vi "Initialize.vi"(8 "error in (no error)":errorcluster, 10 "config path":path, 11 "ThAr in":refnum<class "ThAr.lvclass">) -> (0 "error out":errorcluster, 3 "ThAr out":refnum<class "ThAr.lvclass">)   [LabVIEW 2016, in "ThAr.lvclass"]
uses:
  ThAr.lvclass
  <vilib>/Utility/config.llb/Read Key (Double).vi
  <vilib>/Utility/config.llb/Read Key (U32).vi
  <vilib>/Utility/config.llb/Read Key (String).vi
  Lamp.lvclass
  <vilib>/Utility/config.llb/NI_LVConfig.lvlib
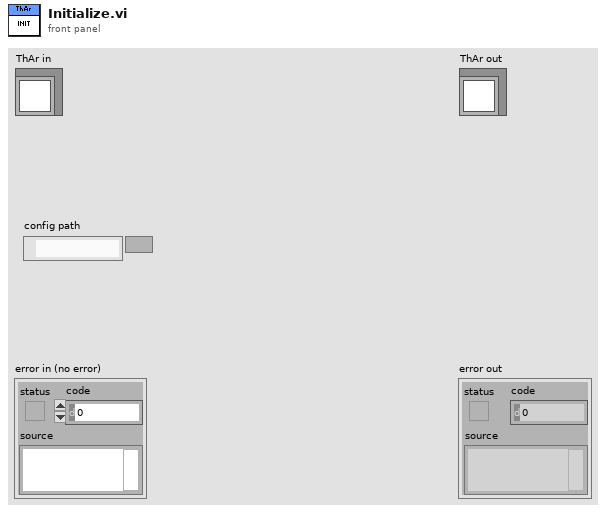
[diagram p1: front panel]
types:
  T1 = typedef "NI_LVConfig.lvlib/Config Data RefNum.ctl" = refnum<k1>
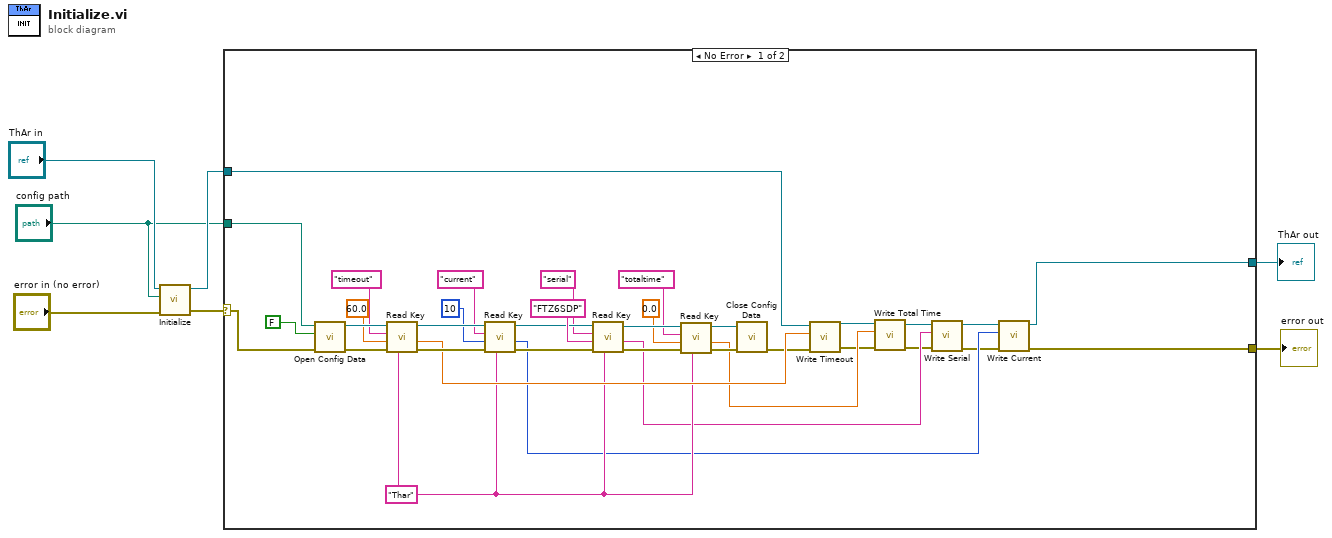
[diagram p0: block diagram]
diagram:
  n1 = call-parent "Initialize.vi"("error in (no error)"="error in (no error)", "config path"="config path", "Lamp in"="ThAr in") -> ("error out"=w4:errorcluster, "Lamp out"=w7:refnum<class "ThAr.lvclass">)  [unwired: 7 in]
  n2 = case shown="No Error" w4 {
    selector: w4 -> [w28 w44]
    tunnel: w7 -> [w29 w45]
    tunnel: "config path" -> [w31 _]
    tunnel: [w9 w44] -> w2
    tunnel: [w8 w45] -> w1
    frame No Error {
      w23 = "Thar" ("section")
      n3 = call <vilib>:"Open Config Data.vi"("error in (no error)"=w28, "create file if necessary (T)"=FALSE, "configuration file path"=w31) -> ("error out"=w36:errorcluster, "refnum"=w42:T1)  [unwired: 6 in, 1 out]
      n4 = call-poly <vilib>:"Read Key.vi"("section"=w23, "error in (no error)"=w36, "default value"=60.0, "key"="timeout" ("element"), "refnum"=w42) -> ("error out"=w37:errorcluster, "value"=w27:dbl, "refnum out"=w41:T1)  [unwired: 3 in, 1 out]
      n5 = call-poly <vilib>:"Read Key.vi"("section"=w23, "error in (no error)"=w37, "default value"=u32 10, "key"="current", "refnum"=w41) -> ("error out"=w34:errorcluster, "value"=w12:u32, "refnum out"=w32:T1)  [unwired: 3 in, 1 out]
      n6 = call-poly <vilib>:"Read Key.vi"("section"=w23, "error in (no error)"=w34, "default value"="FTZ6SDP", "key"="serial", "refnum"=w32) -> ("error out"=w19:errorcluster, "value"=w14:string, "refnum out"=w22:T1)  [unwired: 3 in, 1 out]
      n7 = call-poly <vilib>:"Read Key.vi"("section"=w23, "error in (no error)"=w19, "default value"=0.0, "key"="totaltime", "refnum"=w22) -> ("error out"=w24:errorcluster, "value"=w18:dbl, "refnum out"=w25:T1)  [unwired: 3 in, 1 out]
      n8 = call <vilib>:"Close Config Data.vi"("error in (no error)"=w24, "refnum"=w25) -> ("error out"=w26:errorcluster)  [unwired: 8 in, 1 out]
      n9 = call-dynamic "Write Timeout.vi"("error in (no error)"=w26, "Timeout"=w27, "Lamp in"=w29) -> ("error out"=w17:errorcluster, "Lamp out"=w16:refnum<class "ThAr.lvclass">)  [unwired: 7 in]
      n10 = call-dynamic "Write Total Time.vi"("error in (no error)"=w17, "Total Time"=w18, "Lamp in"=w16) -> ("error out"=w11:errorcluster, "Lamp out"=w15:refnum<class "ThAr.lvclass">)  [unwired: 7 in]
      n11 = call-dynamic "Write Serial.vi"("error in (no error)"=w11, "Serial"=w14, "ThAr in"=w15) -> ("error out"=w10:errorcluster, "ThAr out"=w13:refnum<class "ThAr.lvclass">)  [unwired: 7 in]
      n12 = call-dynamic "Write Current.vi"("error in (no error)"=w10, "current [mA]"=w12, "ThAr in"=w13) -> ("error out"=w9:errorcluster, "ThAr out"=w8:refnum<class "ThAr.lvclass">)  [unwired: 7 in]
    }
    frame Error {
    }
  }
  "error out" <- w2
  "ThAr out" <- w1
